vi "I2C Open Channel.vi"(8 "error in (no error)":errorcluster, 11 "index":u32) -> (0 "error out 2":errorcluster, 3 "handle out 2":u64 format="%0x")   [LabVIEW 2024, in "libMPSSE-I2C.lvlib"]
doc: "FTDI_API FT_STATUS SPI_OpenChannel(uint32 index, FT_HANDLE *handle);"
uses:
  libMPSSE-I2C.lvlib
  subvi/ChannelConfig.ctl
  libmpsse.dll
panel:
  out "handle 2":u64 format="%x"
  out "Return (Init)":u64
  out "Return (open)":u64
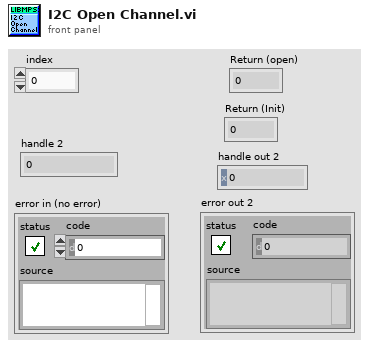
[diagram p1: front panel]
types:
  T1 = typedef "libMPSSE-I2C.lvlib/ChannelConfig.ctl" = cluster{"ClockRate":u32, "LatencyTimer":u8, "Fill1":u8, "Fill 2":u8, "Fill 3":u8, "Options":u32, "Pin":u32, "currentPinState":u16}
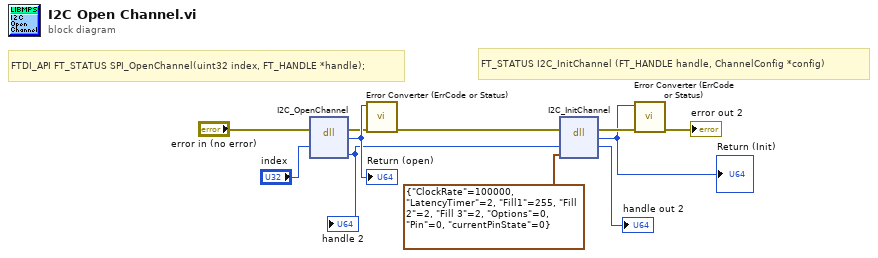
[diagram p0: block diagram]
diagram:
  # "FT_STATUS I2C_InitChannel (FT_HANDLE handle, ChannelConfig *config)"
  # "FTDI_API FT_STATUS SPI_OpenChannel(uint32 index, FT_HANDLE *handle);"
  n1 = dll-call lib="C:/Sandbox/sm_6576_001_RIB_Sequencer/I2C/libmpsse.dll" fn="I2C_OpenChannel"(error in="error in (no error)", "index"="index") -> (error out=w8:errorcluster, "return type"=w11:u64, "handle"=w2:u64)  [unwired: 4 in, 1 out]
  "Return (open)" <- w11
  "handle 2" <- w2
  n2 = call "Error Converter (ErrCode or Status).vi"("error in (no error)"=w8, "error code"=w11) -> ("error out"=w4:errorcluster)  [unwired: 9 in]
  n3 = dll-call lib="C:/Sandbox/sm_6576_001_RIB_Sequencer/I2C/libmpsse.dll" fn="I2C_InitChannel"(error in=w4, "handle"=w2, "config"=T1 {"ClockRate"=100000, "LatencyTimer"=2, "Fill1"=255, "Fill 2"=2, "Fill 3"=2, "Options"=0, "Pin"=0, "currentPinState"=0} ("Channelconfig_t")) -> (error out=w6:errorcluster, "return type"=w3:u64, "handle"=→"handle out 2":u64)  [unwired: 3 in, 1 out]
  "Return (Init)" <- w3
  n4 = call "Error Converter (ErrCode or Status).vi"("error in (no error)"=w6, "error code"=w3) -> ("error out"=→"error out 2":errorcluster)  [unwired: 9 in]
